vi "FIFO Read.vi"(0 "FPGA Ref":T3, 5 "Elements Available":T2, 11 "error in":errorcluster, 12 "Imaging Protocol":T1) -> (4 "FPGA VI Reference Out":T3, 6 "Data arrays cluster":T4, 10 "Elements Remaining (Ch0)":u32, 14 "Image Time Elements Remaining":u32, 15 "error out":errorcluster)   [LabVIEW 2017]
uses:
  Typedefs/Data arrays cluster.ctl
  RIG-SPECIFIC FILES/FPGA Refs/FPGA Ref.ctl
  Acquisition/Typedefs/FIFO elements available.ctl
  Typedefs/Imaging Protocols enum.ctl
  <vilib>/Utility/error.llb/Error Cluster From Error Code.vi
  <vilib>/rvi/errors/niLvFpgaAdjustHostInterfaceError.vi
  <vilib>/rvi/interface/nirviMethod/nirviMethod.xnode
  <vilib>/rvi/errors/niLvFpgaMergeErrorWithErrorCode.vi
  <vilib>/FPGAPlugInAG/Dynamic/niLvFpga_ReadFifo_Dynamic.vi
panel:
  out "Continuous Time Elements Remaining":u32
  out "Ref time Elements Remaining":u32
  out "Elements Remaining (Ch1)":u32
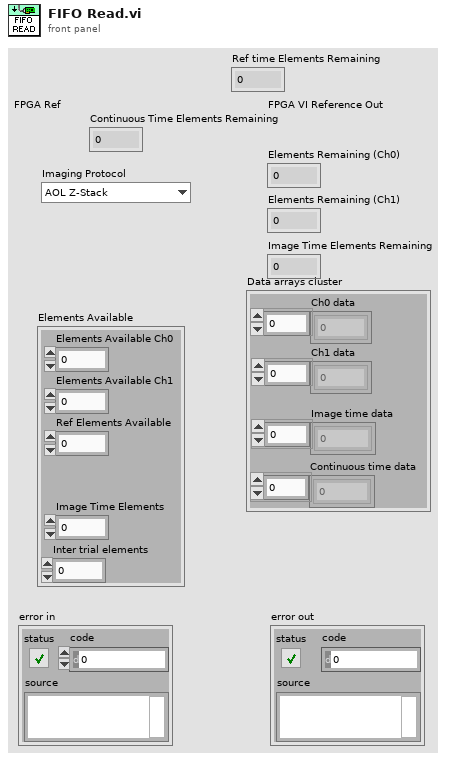
[diagram p1: front panel]
types:
  T1 = typedef "Imaging Protocols enum.ctl" = enum16{"AOL Z-Stack", "Motor Z Stack", "Functional Acquisition", "Single Plane Acquisition", "Volume Acquisition", "Live Imaging", "Live Plane Imaging", "Live Volume Imaging"}
  T2 = typedef "FIFO elements available.ctl" = cluster{"Elements Available Ch0":u32, "Elements Available Ch1":u32, "Ref Elements Available":u32, "Image Time Elements":u32, "Inter trial elements":u32}
  T3 = typedef "FPGA Ref.ctl" = refnum<k20>
  T4 = typedef "Data arrays cluster.ctl" = cluster{"Ch0 data":u32[], "Ch1 data":u32[], "Image time data":u64[], "Continuous time data":u64[]}
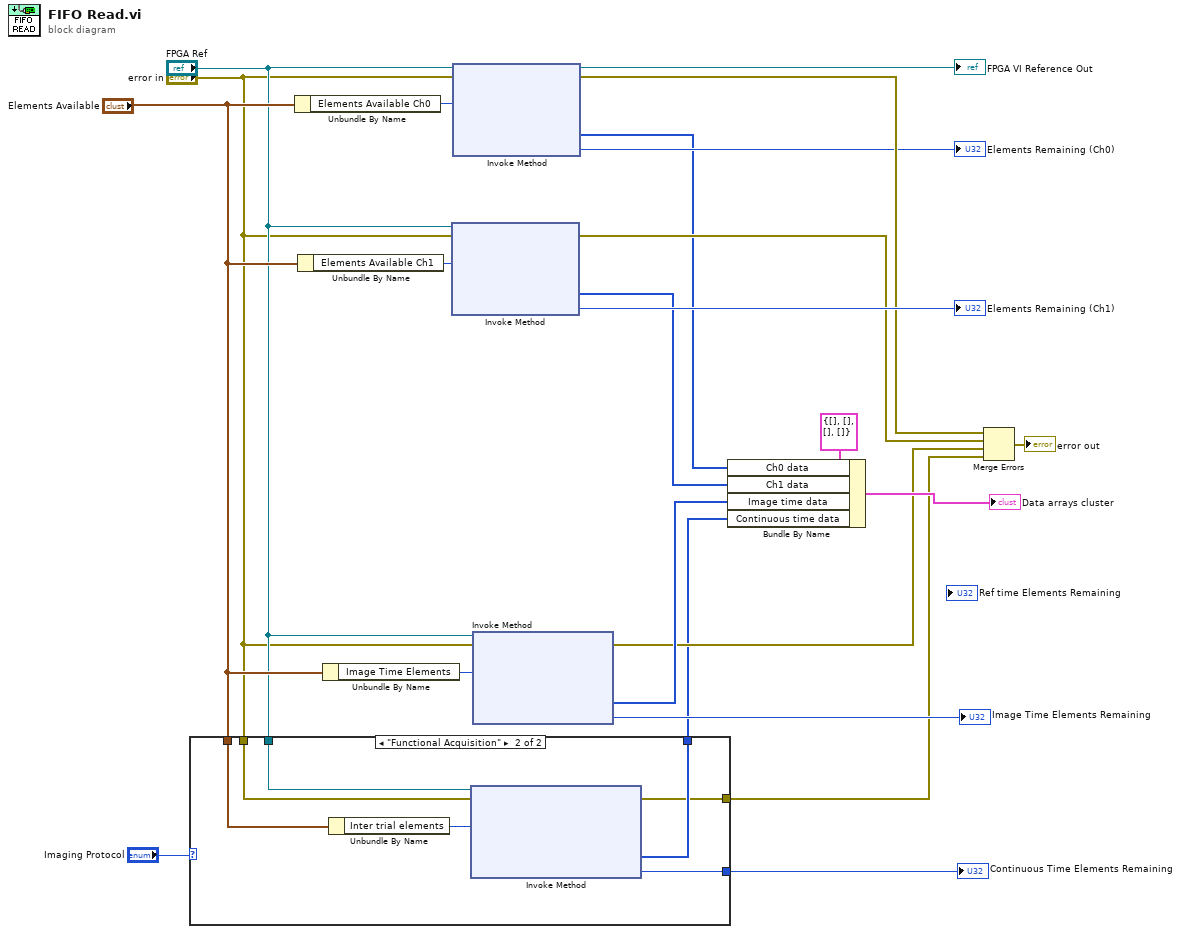
[diagram p0: block diagram]
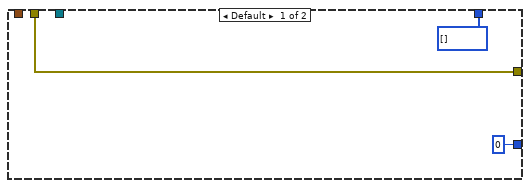
[diagram p2: hidden frame]
diagram:
  n1 = case shown="\"Functional Acquisition\"" "Imaging Protocol" {
    tunnel: "Elements Available" -> [_ w32]
    tunnel: "FPGA Ref" -> [_ w31]
    tunnel: [u64[] [] ("Data") w30] -> w5
    tunnel: [u32 0 ("Elements Remaining") w29] -> w4
    tunnel: [w26 w27] -> w2
    tunnel: "error in" -> [w26 w28]
    frame Default {
    }
    frame "Functional Acquisition" {
      n2 = Unbundle By Name(w32) -> ("Inter trial elements"=w33:u32)
      n3 = xnode ("Invoke Method")("FPGA VI Reference In"=w31, "error in"=w28, "Number of Elements"=w33) -> ("error out"=w27:errorcluster, "Data"=w30:u64[], "Elements Remaining"=w29:u32)  [unwired: 1 in, 1 out]
    }
  }
  "Continuous Time Elements Remaining" <- w4
  n4 = Unbundle By Name("Elements Available") -> ("Elements Available Ch0"=w13:u32)
  n5 = Unbundle By Name("Elements Available") -> ("Elements Available Ch1"=w12:u32)
  n6 = Unbundle By Name("Elements Available") -> ("Image Time Elements"=w11:u32)
  n7 = xnode ("Invoke Method")("FPGA VI Reference In"="FPGA Ref", "error in"="error in", "Number of Elements"=w12) -> ("error out"=w19:errorcluster, "Data"=w15:u32[], "Elements Remaining"=→"Elements Remaining (Ch1)":u32)  [unwired: 1 in, 1 out]
  n8 = xnode ("Invoke Method")("FPGA VI Reference In"="FPGA Ref", "error in"="error in", "Number of Elements"=w13) -> ("FPGA VI Reference Out"=→"FPGA VI Reference Out":T3, "error out"=w20:errorcluster, "Data"=w16:u32[], "Elements Remaining"=→"Elements Remaining (Ch0)":u32)  [unwired: 1 in]
  n9 = xnode ("Invoke Method")("FPGA VI Reference In"="FPGA Ref", "error in"="error in", "Number of Elements"=w11) -> ("error out"=w8:errorcluster, "Data"=w9:u64[], "Elements Remaining"=→"Image Time Elements Remaining":u32)  [unwired: 1 in, 1 out]
  n10 = Bundle By Name(cluster=T4 {"Ch0 data"=[], "Ch1 data"=[], "Image time data"=[], "Continuous time data"=[]} ("Data arrays cluster"), "Ch0 data"=w16, "Ch1 data"=w15, "Image time data"=w9, "Continuous time data"=w5) -> (→"Data arrays cluster":T4)
  n11 = Merge Errors(w20, w19, w8, w2) -> (→"error out":errorcluster)
